vi "Main.vi"() -> ()   [LabVIEW 2017]
uses:
  1. CTL/State.ctl
  <vilib>/Utility/sysdir.llb/System Directory Type.ctl
  <vilib>/Instr/_visa.llb/VISA Configure Serial Port (Instr).vi
panel:
  in  "탭 컨트롤":enum32{"SETTING", "MAIN"}(tab)
  in  "로그인":bool
  in  "비밀번호":string
  in  "ID":string
  in  "COM포트":bool=TRUE
  in  "정지 버튼":bool=TRUE
  in  "PNF ON":bool=TRUE
  in  "데이터 저장":bool=TRUE
  out "시험결과":string
  out "1회시험결과":string
  out "2회시험결과":string
  out "3회시험결과":string
  out "String":string
  out "String 2":string
  out "String 3":string
  in  "VISA resource name":refnum<visa-resource-name> caption="VISA 리소스 이름"
  in  "Radio Buttons":enum32{"Item 0", "Item 1"}(radio)
  # "GUI Setting(KWFI)"
  # "ID"
  # "password"
  # "AUV Pinger TEST"
  # "음파발생기 TEST"
  # "시험 결과"
  # "시험 결과"
  # "1회 시험 데이터"
  # "2회 시험 데이터"
  # "3회 시험 데이터"
  # "1회 시험 결과"
  # "2회 시험 결과"
  # "3회 시험 결과"
  # "1회 시험 결과"
  # "2회 시험 결과"
  # "3회 시험 결과"
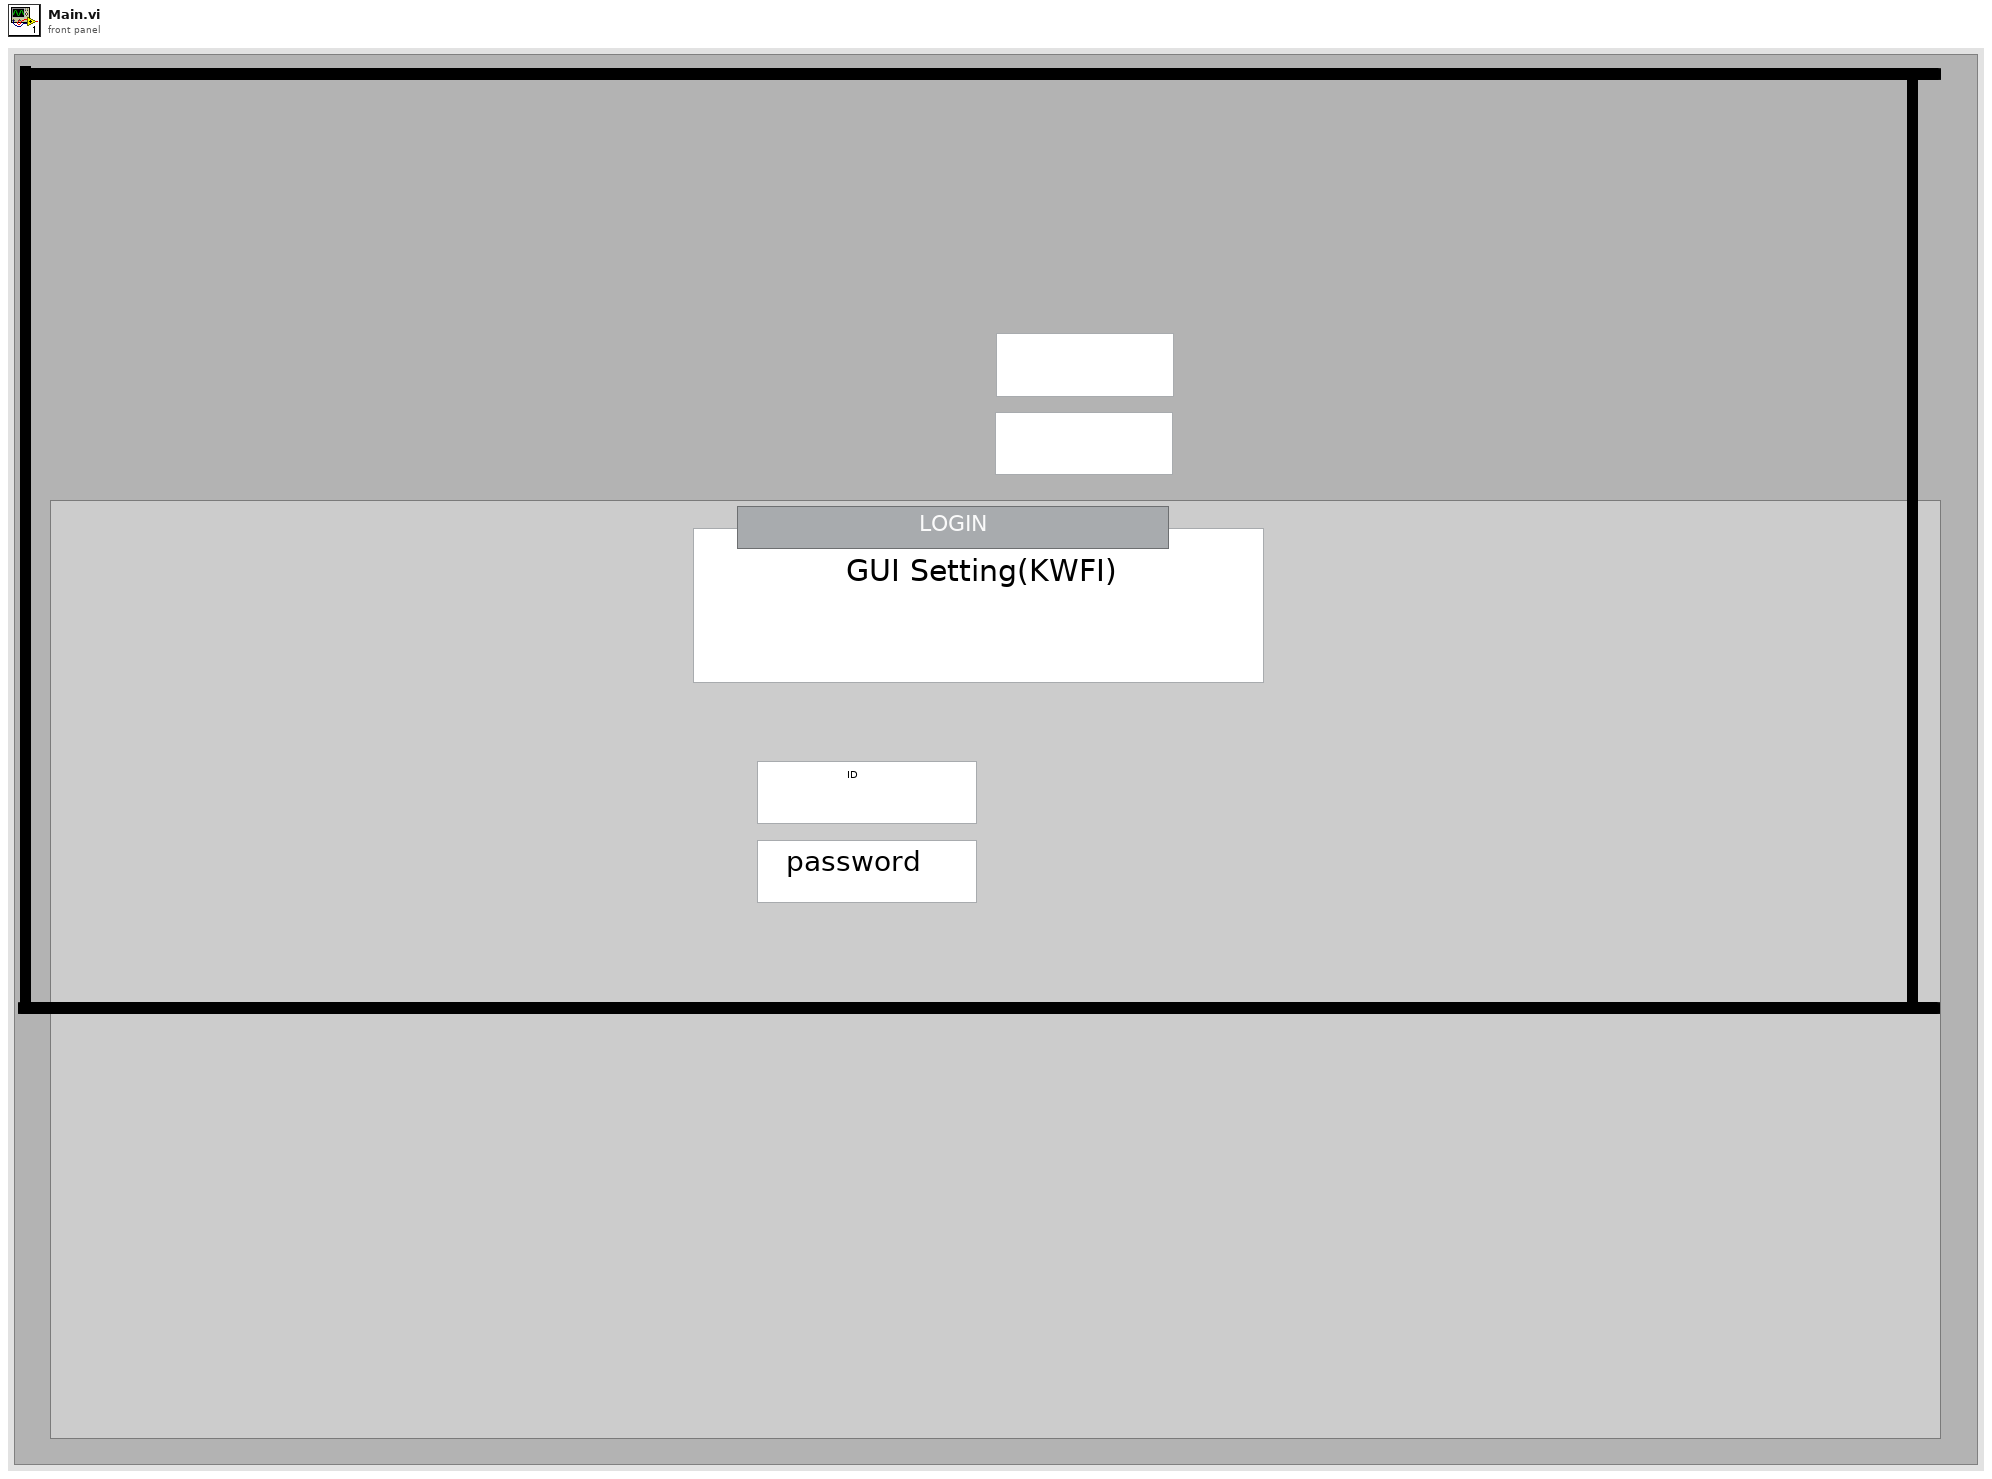
[diagram p1: front panel]
types:
  T1 = cluster{"1회 시험결과":string, "2회 시험결과":string, "3회 시험결과":string, "시험결과":string, "COM 포트":refnum<visa-resource-name>, "카운터":i32, "1회 로그":string, "2회 로그":string, "3회 로그":string, "1회 결과 카운트":i32, "2회 결과 카운트":i32, "3회 결과 카운트":i32, "관리자모드":bool, "1회 데이터":string[], "2회 데이터":string[], "3회 데이터":string[]}
  T2 = typedef "State.ctl" = enum16{"초기화", "시작", "정지", "데이터 저장", "로그인"}
  T3 = enum16{"open", "open or create", "create or replace", "create", "open (read-only)"}
  T4 = typedef "System Directory Type.ctl" = i32
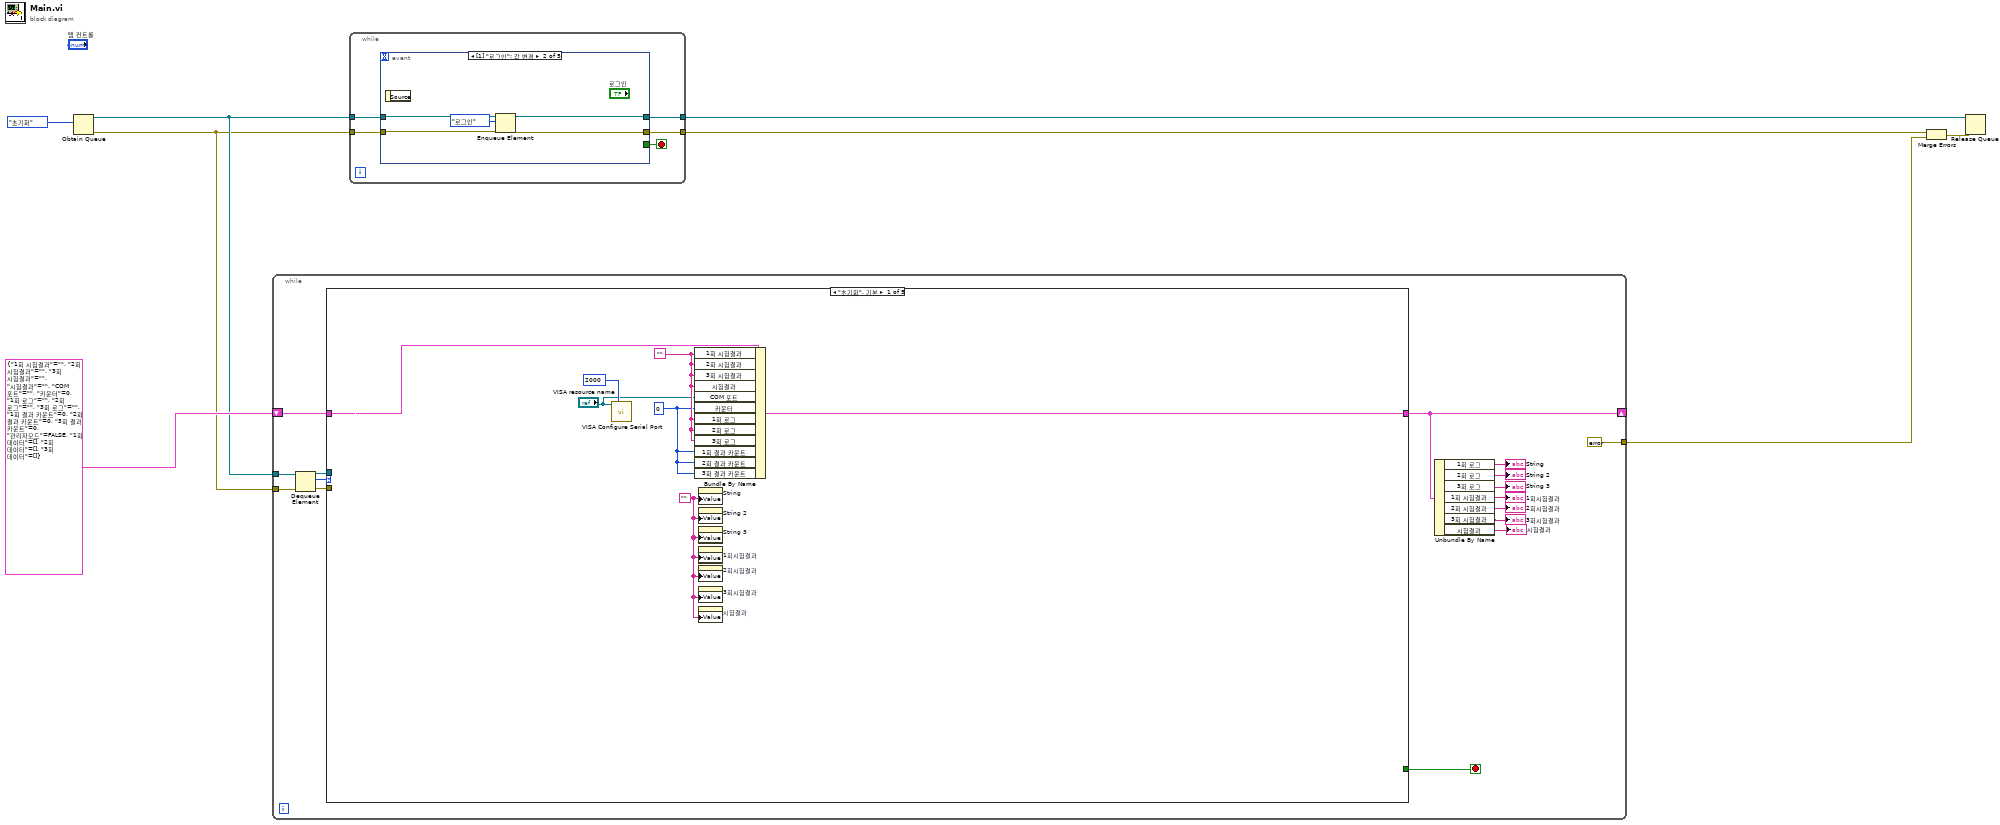
[diagram p0: block diagram]
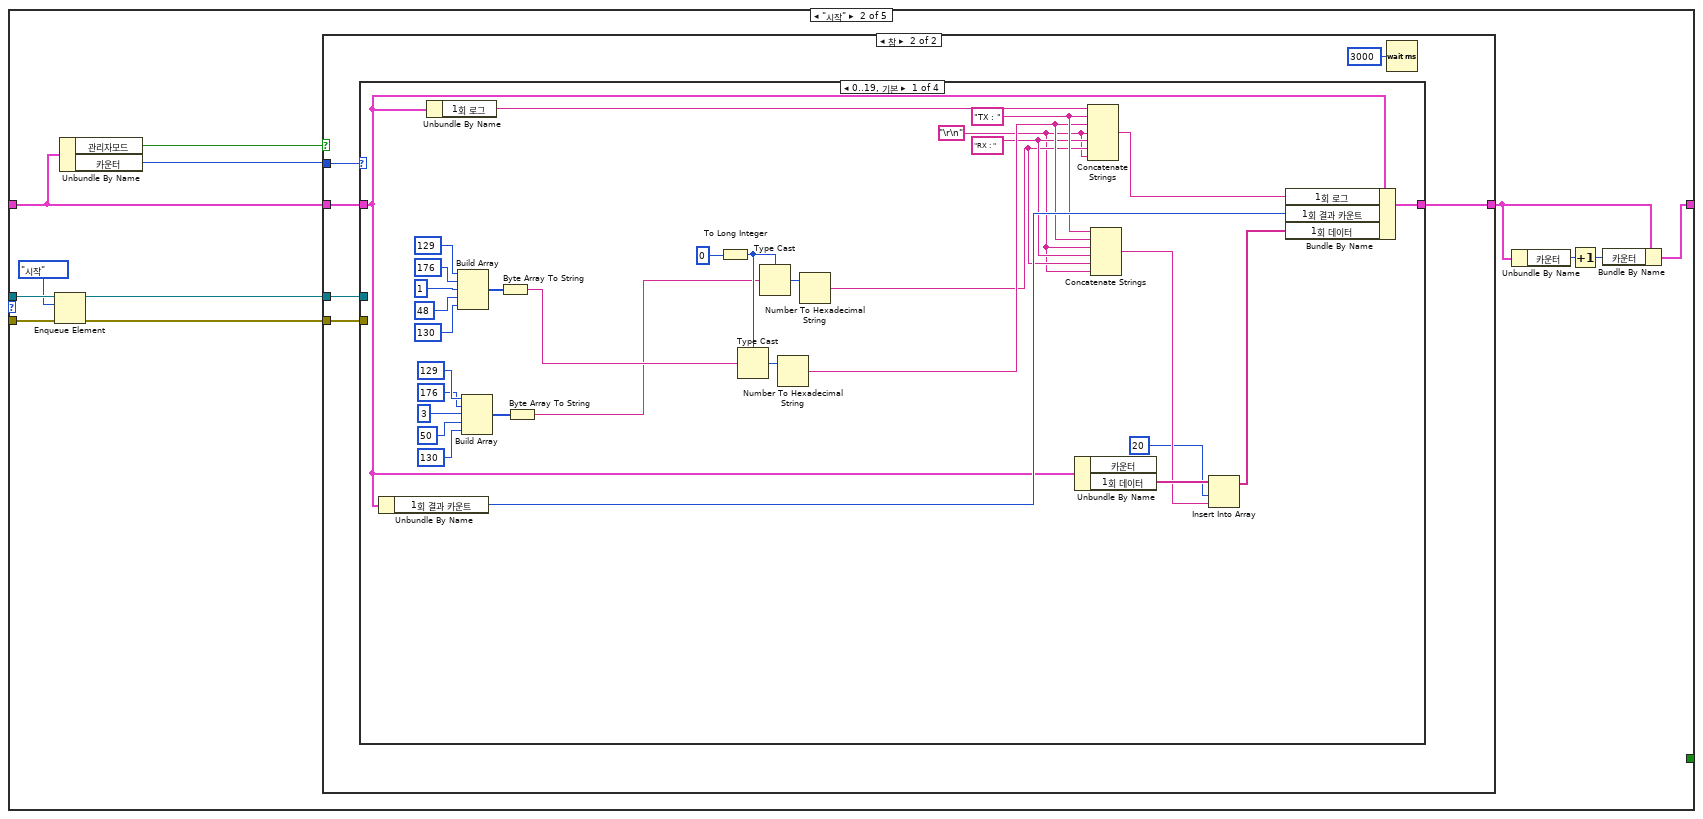
[diagram p2: hidden frame]
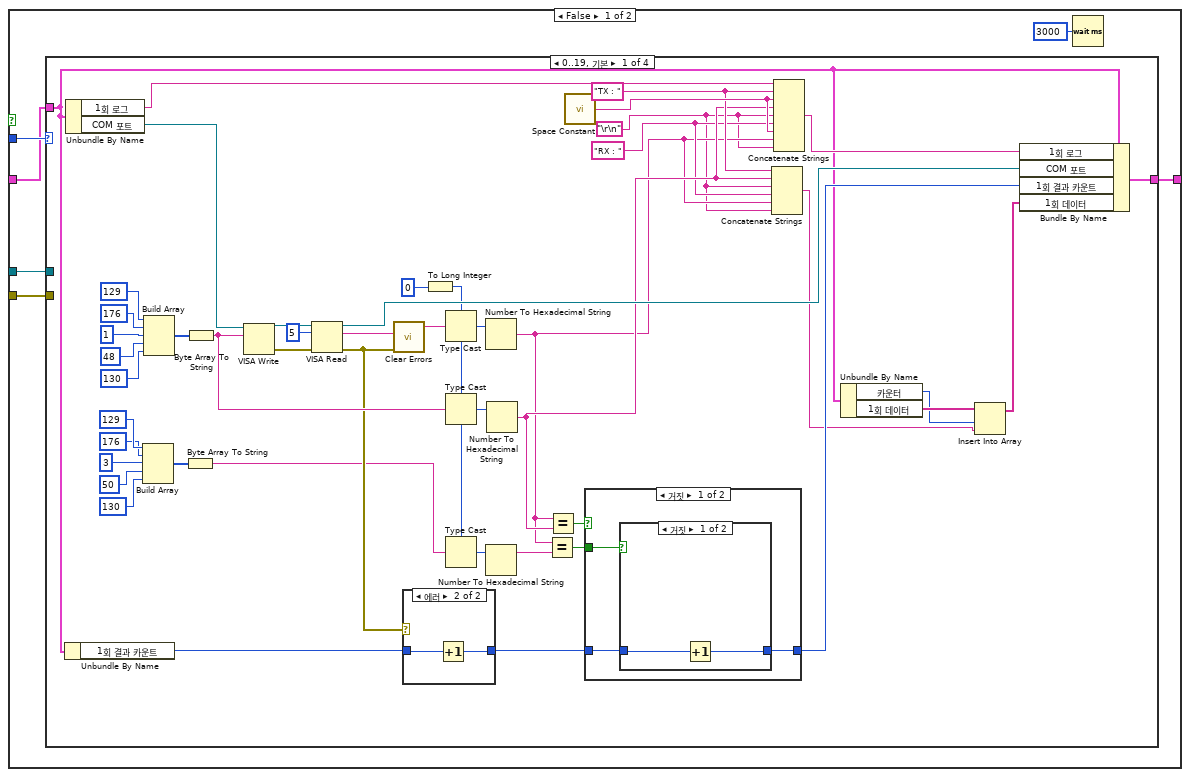
[diagram p3: hidden frame]
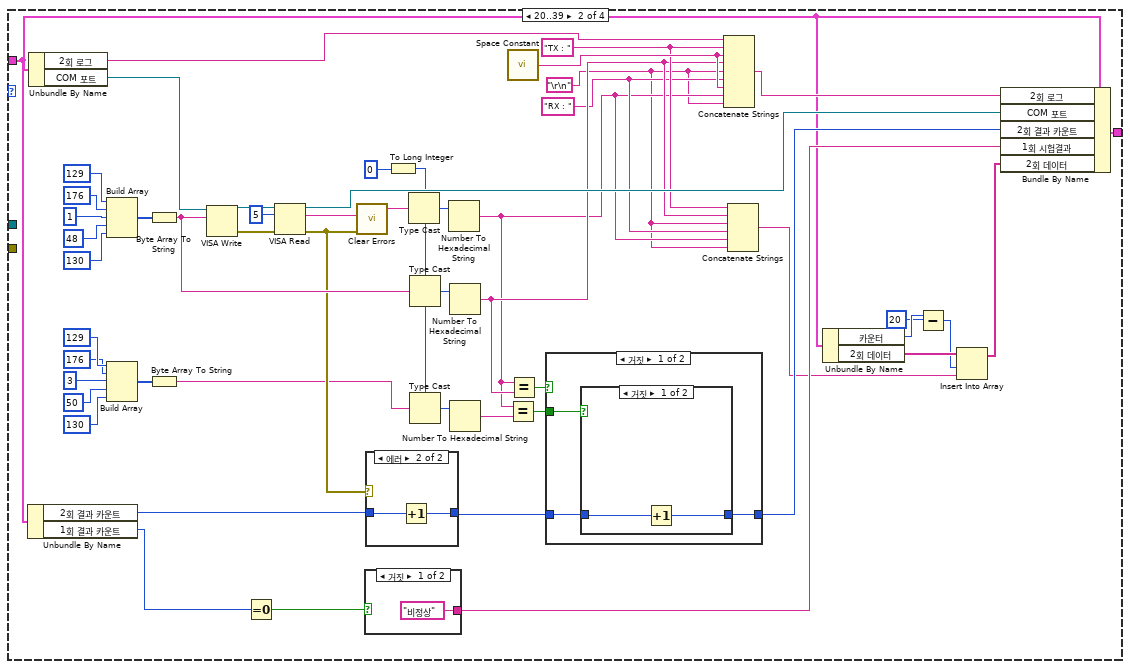
[diagram p7: hidden frame]
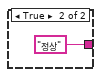
[diagram p10: hidden frame]
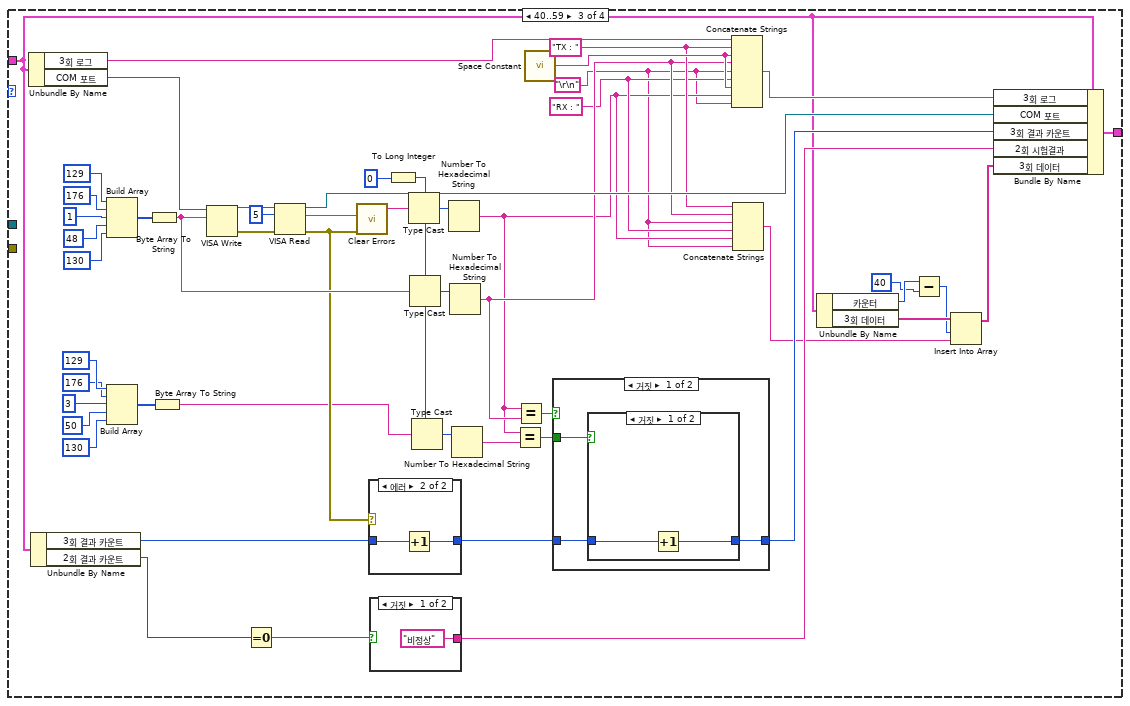
[diagram p12: hidden frame]
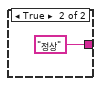
[diagram p15: hidden frame]
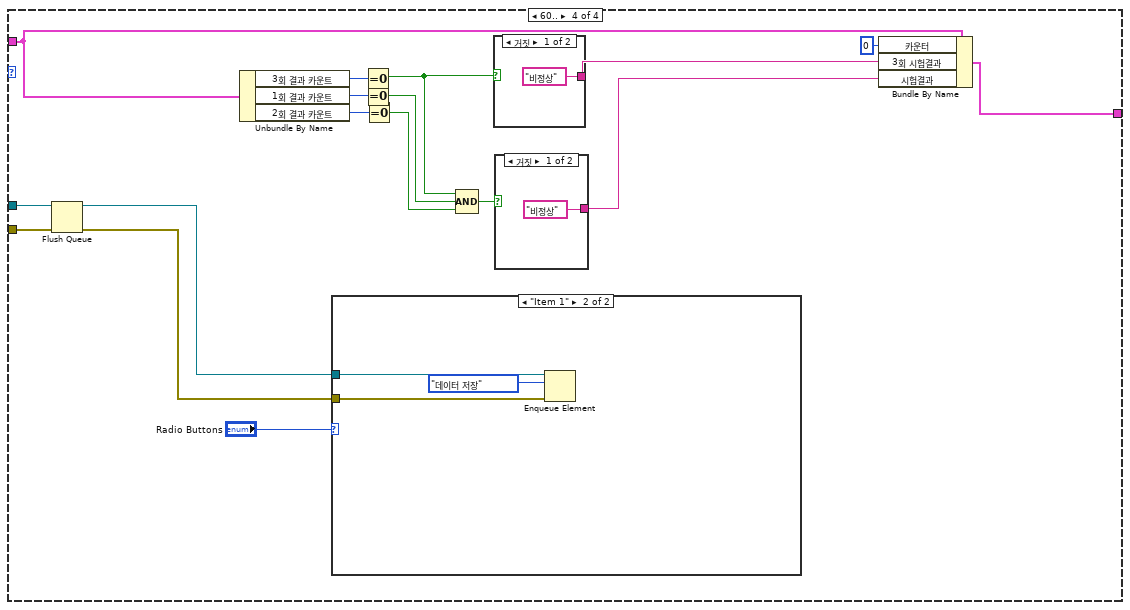
[diagram p17: hidden frame]
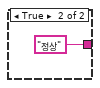
[diagram p19: hidden frame]
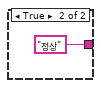
[diagram p20: hidden frame]
diagram:
  n1 = Obtain Queue(element data type=State."초기화") -> (queue out=w2:refnum<queue>, error out=w1:errorcluster)  [unwired: 4 in, 1 out]
  n2 = while {
    tunnel: w2 -> [w20]
    tunnel: w1 -> [w24]
    tunnel: [errorcluster {"status"=FALSE, "code"=0, "source"=""} ("에러 상수")] -> w6
    shift-right: [w9] -> _
    shift-left: T1 {"1회 시험결과"="", "2회 시험결과"="", "3회 시험결과"="", "시험결과"="", "COM 포트"="", "카운터"=0, "1회 로그"="", "2회 로그"="", "3회 로그"="", "1회 결과 카운트"=0, "2회 결과 카운트"=0, "3회 결과 카운트"=0, "관리자모드"=FALSE, "1회 데이터"=[], "2회 데이터"=[], "3회 데이터"=[]} -> [w21]
    stop <- w23 stop-if-true
    n3 = Dequeue Element(queue=w20, error in (no error)=w24) -> (queue out=w18:refnum<queue>, element=w19:T2, error out=w17:errorcluster)  [unwired: 1 in, 1 out]
    n4 = case shown="\"초기화\", 기본" w19 {
      tunnel: [_ _ TRUE _ _] -> w23
      tunnel: w21 -> [w31 w36 w386 w406 w440]
      tunnel: w18 -> [_ w42 _ w430 _]
      tunnel: w17 -> [_ w41 _ w429 _]
      tunnel: [w27 w32 w386 w406 w439] -> w9
      frame "초기화", Default {
        w28 = 0
        w29 = ""
        w30 = ""
        n5 = call-poly "VISA Configure Serial Port"("VISA resource name"="VISA resource name", "timeout (10sec)"=u32 2000) -> ()  [unwired: 12 in, 2 out]
        n6 = Bundle By Name(cluster=w31, "1회 시험결과"=w29, "2회 시험결과"=w29, "3회 시험결과"=w29, "시험결과"=w29, "COM 포트"="VISA resource name", "카운터"=w28, "1회 로그"=w29, "2회 로그"=w29, "3회 로그"=w29, "1회 결과 카운트"=w28, "2회 결과 카운트"=w28, "3회 결과 카운트"=w28) -> (w27:T1)
        n7 = property on="String" class="Str"("Value"=w30) -> ()  [unwired: 2 in, 2 out]
        n8 = property on="String 2" class="Str"("Value"=w30) -> ()  [unwired: 2 in, 2 out]
        n9 = property on="String 3" class="Str"("Value"=w30) -> ()  [unwired: 2 in, 2 out]
        n10 = property on="1회시험결과" class="Str"("Value"=w30) -> ()  [unwired: 2 in, 2 out]
        n11 = property on="2회시험결과" class="Str"("Value"=w30) -> ()  [unwired: 2 in, 2 out]
        n12 = property on="3회시험결과" class="Str"("Value"=w30) -> ()  [unwired: 2 in, 2 out]
        n13 = property on="시험결과" class="Str"("Value"=w30) -> ()  [unwired: 2 in, 2 out]
      }
      frame "시작" {
        n14 = Enqueue Element(queue=w42, element=State."시작", error in (no error)=w41) -> (queue out=w39:refnum<queue>, error out=w38:errorcluster)  [unwired: 1 in, 1 out]
        n15 = Unbundle By Name(w36) -> ("관리자모드"=w37:bool, "카운터"=w43:i32)
        n16 = case shown="참" w37 {
          tunnel: w43 -> [w49 w261]
          tunnel: w39 -> [w48 w260]
          tunnel: w38 -> [w47 w259]
          tunnel: [w45 w257] -> w33
          tunnel: w36 -> [w44 w256]
          frame False {
            n17 = case shown="0..19, 기본" w49 {
              tunnel: w44 -> [w54 w116 w179 w246]
              tunnel: [w95 w156 w219 w247] -> w45
              tunnel: w48 -> [_ _ _ w243]
              tunnel: w47 -> [_ _ _ w242]
              frame 0..19, Default {
                w57 = "RX : "
                w55 = "\r\n"
                w59 = "TX : "
                n18 = Unbundle By Name(w54) -> ("1회 결과 카운트"=w76:i32)
                n19 = Unbundle By Name(w54) -> ("1회 로그"=w82:string, "COM 포트"=w81:refnum<visa-resource-name>)
                n20 = Build Array(129, 176, 3, 50, 130) -> (w74:i32[])
                n21 = Build Array(129, 176, 1, 48, 130) -> (w86:i32[])
                n22 = Byte Array To String(unsigned byte array=w74) -> (string=w67:string)
                n23 = Byte Array To String(unsigned byte array=w86) -> (string=w80:string)
                n24 = VISA Write(VISA resource name=w81, write buffer=w80) -> (VISA resource name out=w94:refnum<visa-resource-name>, error out=w92:errorcluster)  [unwired: 1 in, 1 out]
                n25 = VISA Read(VISA resource name=w94, byte count=u32 5 ("바이트 카운트"), error in (no error)=w92) -> (VISA resource name out=w79:refnum<visa-resource-name>, read buffer=w85:string, error out=w77:errorcluster)  [unwired: 1 out]
                n26 = call <vilib>:"Clear Errors.vi"("error in (no error)"=w77) -> ()  [unwired: 5 in, 2 out]
                n27 = case shown="에러" w77 {
                  tunnel: [w103 w105] -> w63
                  tunnel: w76 -> [w103 w104]
                  frame No Error {
                  }
                  frame Error {
                    n28 = Increment(x=w104) -> (x+1=w105:i32)
                  }
                }
                n29 = To Long Integer(number=0 ("숫자")) -> (32bit integer=w68:i32)
                n30 = Type Cast(type=w68, x=w85) -> (*(type *) &x=w84:i32)
                n31 = Type Cast(type=w68, x=w80) -> (*(type *) &x=w78:i32)
                n32 = Type Cast(type=w68, x=w67) -> (*(type *) &x=w66:i32)
                n33 = Number To Hexadecimal String(2:w84) -> (0:w56:string)  [unwired: 1 in]
                n34 = Number To Hexadecimal String(2:w66) -> (0:w64:string)  [unwired: 1 in]
                n35 = Number To Hexadecimal String(2:w78) -> (0:w58:string)  [unwired: 1 in]
                n36 = Equal?(x=w56, y=w64) -> (x = y?=w65:bool)
                n37 = Equal?(x=w56, y=w58) -> (x = y?=w75:bool)
                n38 = call <vilib>:"Space Constant.vi"() -> ("String"=w61:string)
                n39 = case shown="거짓" w75 {
                  tunnel: w65 -> [w98 _]
                  tunnel: w63 -> [w97 w102]
                  tunnel: [w96 w102] -> w62
                  frame False {
                    n40 = case shown="거짓" w98 {
                      tunnel: w97 -> [w100 w101]
                      tunnel: [w99 w101] -> w96
                      frame False {
                        n41 = Increment(x=w100) -> (x+1=w99:i32)
                      }
                      frame True {
                      }
                    }
                  }
                  frame True {
                  }
                }
                n42 = Concatenate Strings(w59, w58, w55, w57, w56, w55) -> (w52:string)
                n43 = Concatenate Strings(w82, w59, w61, w58, w55, w57, w61, w56, w55) -> (w60:string)
                n44 = Unbundle By Name(w54) -> ("카운터"=w50:i32, "1회 데이터"=w53:string[])
                n45 = Insert Into Array(array=w53, index=w50, new element=w52) -> (w51:string[])
                n46 = Bundle By Name(cluster=w54, "1회 로그"=w60, "COM 포트"=w79, "1회 결과 카운트"=w62, "1회 데이터"=w51) -> (w95:T1)
              }
              frame 20..39 {
                w113 = "RX : "
                w111 = "\r\n"
                w115 = "TX : "
                n47 = Unbundle By Name(w116) -> ("2회 결과 카운트"=w138:i32, "1회 결과 카운트"=w137:i32)
                n48 = Unbundle By Name(w116) -> ("2회 로그"=w120:string, "COM 포트"=w143:refnum<visa-resource-name>)
                n49 = Build Array(129, 176, 1, 48, 130) -> (w147:i32[])
                n50 = Build Array(129, 176, 3, 50, 130) -> (w132:i32[])
                n51 = Byte Array To String(unsigned byte array=w147) -> (string=w142:string)
                n52 = Byte Array To String(unsigned byte array=w132) -> (string=w124:string)
                n53 = VISA Write(VISA resource name=w143, write buffer=w142) -> (VISA resource name out=w155:refnum<visa-resource-name>, error out=w153:errorcluster)  [unwired: 1 in, 1 out]
                n54 = Equal To 0?(x=w137) -> (x = 0?=w136:bool)
                n55 = VISA Read(VISA resource name=w155, byte count=u32 5 ("바이트 카운트"), error in (no error)=w153) -> (VISA resource name out=w141:refnum<visa-resource-name>, read buffer=w146:string, error out=w139:errorcluster)  [unwired: 1 out]
                n56 = call <vilib>:"Clear Errors.vi"("error in (no error)"=w139) -> ()  [unwired: 5 in, 2 out]
                n57 = case shown="거짓" w136 {
                  tunnel: ["비정상" "정상"] -> w135
                  frame False {
                  }
                  frame True {
                  }
                }
                n58 = case shown="에러" w139 {
                  tunnel: [w166 w168] -> w122
                  tunnel: w138 -> [w166 w167]
                  frame No Error {
                  }
                  frame Error {
                    n59 = Increment(x=w167) -> (x+1=w168:i32)
                  }
                }
                n60 = To Long Integer(number=0 ("숫자")) -> (32bit integer=w125:i32)
                n61 = Type Cast(type=w125, x=w146) -> (*(type *) &x=w145:i32)
                n62 = Type Cast(type=w125, x=w142) -> (*(type *) &x=w140:i32)
                n63 = Type Cast(type=w125, x=w124) -> (*(type *) &x=w126:i32)
                n64 = Number To Hexadecimal String(2:w145) -> (0:w112:string)  [unwired: 1 in]
                n65 = Number To Hexadecimal String(2:w140) -> (0:w114:string)  [unwired: 1 in]
                n66 = Number To Hexadecimal String(2:w126) -> (0:w123:string)  [unwired: 1 in]
                n67 = call <vilib>:"Space Constant.vi"() -> ("String"=w119:string)
                n68 = Equal?(x=w112, y=w123) -> (x = y?=w133:bool)
                n69 = Equal?(x=w112, y=w114) -> (x = y?=w134:bool)
                n70 = case shown="거짓" w134 {
                  tunnel: w133 -> [w159 _]
                  tunnel: w122 -> [w158 w163]
                  tunnel: [w157 w163] -> w121
                  frame False {
                    n71 = case shown="거짓" w159 {
                      tunnel: w158 -> [w161 w162]
                      tunnel: [w160 w162] -> w157
                      frame False {
                        n72 = Increment(x=w161) -> (x+1=w160:i32)
                      }
                      frame True {
                      }
                    }
                  }
                  frame True {
                  }
                }
                n73 = Concatenate Strings(w120, w115, w119, w114, w111, w113, w119, w112, w111) -> (w118:string)
                n74 = Concatenate Strings(w115, w114, w111, w113, w112, w111) -> (w110:string)
                n75 = Unbundle By Name(w116) -> ("카운터"=w108:i32, "2회 데이터"=w117:string[])
                n76 = Subtract(x=w108, y=20) -> (x-y=w106:i32)
                n77 = Insert Into Array(array=w117, index=w106, new element=w110) -> (w109:string[])
                n78 = Bundle By Name(cluster=w116, "2회 로그"=w118, "COM 포트"=w141, "2회 결과 카운트"=w121, "1회 시험결과"=w135, "2회 데이터"=w109) -> (w156:T1)
              }
              frame 40..59 {
                w176 = "RX : "
                w174 = "\r\n"
                w178 = "TX : "
                n79 = Unbundle By Name(w179) -> ("3회 로그"=w183:string, "COM 포트"=w206:refnum<visa-resource-name>)
                n80 = Unbundle By Name(w179) -> ("3회 결과 카운트"=w201:i32, "2회 결과 카운트"=w200:i32)
                n81 = Build Array(129, 176, 1, 48, 130) -> (w210:i32[])
                n82 = Build Array(129, 176, 3, 50, 130) -> (w195:i32[])
                n83 = Byte Array To String(unsigned byte array=w210) -> (string=w205:string)
                n84 = Byte Array To String(unsigned byte array=w195) -> (string=w187:string)
                n85 = VISA Write(VISA resource name=w206, write buffer=w205) -> (VISA resource name out=w218:refnum<visa-resource-name>, error out=w216:errorcluster)  [unwired: 1 in, 1 out]
                n86 = Equal To 0?(x=w200) -> (x = 0?=w199:bool)
                n87 = VISA Read(VISA resource name=w218, byte count=u32 5 ("바이트 카운트"), error in (no error)=w216) -> (VISA resource name out=w204:refnum<visa-resource-name>, read buffer=w209:string, error out=w202:errorcluster)  [unwired: 1 out]
                n88 = call <vilib>:"Clear Errors.vi"("error in (no error)"=w202) -> ()  [unwired: 5 in, 2 out]
                n89 = case shown="에러" w202 {
                  tunnel: [w229 w231] -> w185
                  tunnel: w201 -> [w229 w230]
                  frame No Error {
                  }
                  frame Error {
                    n90 = Increment(x=w230) -> (x+1=w231:i32)
                  }
                }
                n91 = case shown="거짓" w199 {
                  tunnel: ["비정상" "정상"] -> w198
                  frame False {
                  }
                  frame True {
                  }
                }
                n92 = To Long Integer(number=0 ("숫자")) -> (32bit integer=w188:i32)
                n93 = Type Cast(type=w188, x=w209) -> (*(type *) &x=w208:i32)
                n94 = Type Cast(type=w188, x=w205) -> (*(type *) &x=w203:i32)
                n95 = Type Cast(type=w188, x=w187) -> (*(type *) &x=w189:i32)
                n96 = Number To Hexadecimal String(2:w208) -> (0:w175:string)  [unwired: 1 in]
                n97 = Number To Hexadecimal String(2:w203) -> (0:w177:string)  [unwired: 1 in]
                n98 = Number To Hexadecimal String(2:w189) -> (0:w186:string)  [unwired: 1 in]
                n99 = Equal?(x=w175, y=w186) -> (x = y?=w196:bool)
                n100 = Equal?(x=w175, y=w177) -> (x = y?=w197:bool)
                n101 = call <vilib>:"Space Constant.vi"() -> ("String"=w182:string)
                n102 = case shown="거짓" w197 {
                  tunnel: w196 -> [w222 _]
                  tunnel: w185 -> [w221 w226]
                  tunnel: [w220 w226] -> w184
                  frame False {
                    n103 = case shown="거짓" w222 {
                      tunnel: w221 -> [w224 w225]
                      tunnel: [w223 w225] -> w220
                      frame False {
                        n104 = Increment(x=w224) -> (x+1=w223:i32)
                      }
                      frame True {
                      }
                    }
                  }
                  frame True {
                  }
                }
                n105 = Concatenate Strings(w183, w178, w182, w177, w174, w176, w182, w175, w174) -> (w181:string)
                n106 = Concatenate Strings(w178, w177, w174, w176, w175, w174) -> (w173:string)
                n107 = Unbundle By Name(w179) -> ("카운터"=w171:i32, "3회 데이터"=w180:string[])
                n108 = Subtract(x=w171, y=40) -> (x-y=w169:i32)
                n109 = Insert Into Array(array=w180, index=w169, new element=w173) -> (w172:string[])
                n110 = Bundle By Name(cluster=w179, "3회 로그"=w181, "COM 포트"=w204, "3회 결과 카운트"=w184, "2회 시험결과"=w198, "3회 데이터"=w172) -> (w219:T1)
              }
              frame 60.. {
                n111 = Flush Queue(queue=w243, error in (no error)=w242) -> (queue out=w233:refnum<queue>, error out=w232:errorcluster)  [unwired: 1 out]
                n112 = Unbundle By Name(w246) -> ("3회 결과 카운트"=w245:i32, "1회 결과 카운트"=w241:i32, "2회 결과 카운트"=w240:i32)
                n113 = case shown="\"Item 1\"" "Radio Buttons" {
                  tunnel: w233 -> [_ w251]
                  tunnel: w232 -> [_ w250]
                  frame "Item 0", Default {
                  }
                  frame "Item 1" {
                    n114 = Enqueue Element(queue=w251, element=State."데이터 저장", error in (no error)=w250) -> ()  [unwired: 1 in, 3 out]
                  }
                }
                n115 = Equal To 0?(x=w245) -> (x = 0?=w239:bool)
                n116 = Equal To 0?(x=w241) -> (x = 0?=w238:bool)
                n117 = Equal To 0?(x=w240) -> (x = 0?=w237:bool)
                n118 = Compound Arithmetic op=AND(w239, w238, w237) -> (w236:bool)
                n119 = case shown="거짓" w239 {
                  tunnel: ["비정상" "정상"] -> w244
                  frame False {
                  }
                  frame True {
                  }
                }
                n120 = case shown="거짓" w236 {
                  tunnel: ["비정상" "정상"] -> w235
                  frame False {
                  }
                  frame True {
                  }
                }
                n121 = Bundle By Name(cluster=w246, "카운터"=0, "3회 시험결과"=w244, "시험결과"=w235) -> (w247:T1)
              }
            }
            n122 = Wait (ms)(milliseconds to wait=u32 3000 ("대기 시간 (ms)")) -> ()  [unwired: 1 out]
          }
          frame True {
            n123 = case shown="0..19, 기본" w261 {
              tunnel: w256 -> [w264 w297 w336 w377]
              tunnel: [w292 w329 w368 w378] -> w257
              tunnel: w260 -> [_ _ _ w373]
              tunnel: w259 -> [_ _ _ w372]
              frame 0..19, Default {
                w268 = "RX : "
                w270 = "TX : "
                w266 = "\r\n"
                n124 = Unbundle By Name(w264) -> ("1회 결과 카운트"=w279:i32)
                n125 = Unbundle By Name(w264) -> ("1회 로그"=w283:string)
                n126 = Build Array(129, 176, 1, 48, 130) -> (w286:i32[])
                n127 = Build Array(129, 176, 3, 50, 130) -> (w278:i32[])
                n128 = Byte Array To String(unsigned byte array=w286) -> (string=w280:string)
                n129 = Byte Array To String(unsigned byte array=w278) -> (string=w272:string)
                n130 = To Long Integer(number=0 ("숫자")) -> (32bit integer=w282:i32)
                n131 = Type Cast(type=w282, x=w280) -> (*(type *) &x=w281:i32)
                n132 = Type Cast(type=w282, x=w272) -> (*(type *) &x=w285:i32)
                n133 = Number To Hexadecimal String(2:w281) -> (0:w269:string)  [unwired: 1 in]
                n134 = Number To Hexadecimal String(2:w285) -> (0:w267:string)  [unwired: 1 in]
                n135 = Unbundle By Name(w264) -> ("1회 데이터"=w271:string[])  [unwired: 1 out]
                n136 = Concatenate Strings(w283, w270, w269, w266, w268, w267, w266) -> (w293:string)
                n137 = Concatenate Strings(w270, w269, w266, w268, w267, w266) -> (w265:string)
                n138 = Insert Into Array(array=w271, index=20, new element=w265) -> (w263:string[])
                n139 = Bundle By Name(cluster=w264, "1회 로그"=w293, "1회 결과 카운트"=w279, "1회 데이터"=w263) -> (w292:T1)
              }
              frame 20..39 {
                w302 = "RX: "
                w304 = "TX: "
                w300 = "\r\n"
                n140 = Unbundle By Name(w297) -> ("2회 결과 카운트"=w314:i32, "1회 결과 카운트"=w317:i32)
                n141 = Unbundle By Name(w297) -> ("2회 로그"=w320:string)
                n142 = Build Array(129, 176, 3, 50, 130) -> (w312:i32[])
                n143 = Build Array(129, 176, 1, 48, 130) -> (w323:i32[])
                n144 = Byte Array To String(unsigned byte array=w323) -> (string=w313:string)
                n145 = Byte Array To String(unsigned byte array=w312) -> (string=w306:string)
                n146 = Equal To 0?(x=w317) -> (x = 0?=w316:bool)
                n147 = case shown="거짓" w316 {
                  tunnel: ["비정상" "정상"] -> w315
                  frame False {
                  }
                  frame True {
                  }
                }
                n148 = To Long Integer(number=0 ("숫자")) -> (32bit integer=w319:i32)
                n149 = Type Cast(type=w319, x=w306) -> (*(type *) &x=w322:i32)
                n150 = Type Cast(type=w319, x=w313) -> (*(type *) &x=w318:i32)
                n151 = Number To Hexadecimal String(2:w322) -> (0:w301:string)  [unwired: 1 in]
                n152 = Number To Hexadecimal String(2:w318) -> (0:w303:string)  [unwired: 1 in]
                n153 = Unbundle By Name(w297) -> ("카운터"=w296:i32, "2회 데이터"=w305:string[])
                n154 = Concatenate Strings(w320, w304, w303, w300, w302, w301, w300) -> (w330:string)
                n155 = Concatenate Strings(w304, w303, w300, w302, w301, w300) -> (w299:string)
                n156 = Subtract(x=w296, y=20) -> (x-y=w294:i32)
                n157 = Insert Into Array(array=w305, index=w294, new element=w299) -> (w298:string[])
                n158 = Bundle By Name(cluster=w297, "2회 로그"=w330, "2회 결과 카운트"=w314, "1회 시험결과"=w315, "2회 데이터"=w298) -> (w329:T1)
              }
              frame 40..59 {
                w341 = "RX: "
                w343 = "TX: "
                w339 = "\r\n"
                n159 = Unbundle By Name(w336) -> ("3회 결과 카운트"=w353:i32, "2회 결과 카운트"=w356:i32)
                n160 = Unbundle By Name(w336) -> ("3회 로그"=w359:string)
                n161 = Build Array(129, 176, 3, 50, 130) -> (w351:i32[])
                n162 = Build Array(129, 176, 1, 48, 130) -> (w362:i32[])
                n163 = Byte Array To String(unsigned byte array=w351) -> (string=w345:string)
                n164 = Byte Array To String(unsigned byte array=w362) -> (string=w352:string)
                n165 = Equal To 0?(x=w356) -> (x = 0?=w355:bool)
                n166 = case shown="거짓" w355 {
                  tunnel: ["비정상" "정상"] -> w354
                  frame False {
                  }
                  frame True {
                  }
                }
                n167 = To Long Integer(number=0 ("숫자")) -> (32bit integer=w358:i32)
                n168 = Type Cast(type=w358, x=w345) -> (*(type *) &x=w361:i32)
                n169 = Type Cast(type=w358, x=w352) -> (*(type *) &x=w357:i32)
                n170 = Number To Hexadecimal String(2:w361) -> (0:w340:string)  [unwired: 1 in]
                n171 = Number To Hexadecimal String(2:w357) -> (0:w342:string)  [unwired: 1 in]
                n172 = Unbundle By Name(w336) -> ("카운터"=w335:i32, "3회 데이터"=w344:string[])
                n173 = Concatenate Strings(w359, w343, w342, w339, w341, w340, w339) -> (w369:string)
                n174 = Concatenate Strings(w343, w342, w339, w341, w340, w339) -> (w338:string)
                n175 = Subtract(x=w335, y=40) -> (x-y=w333:i32)
                n176 = Insert Into Array(array=w344, index=w333, new element=w338) -> (w337:string[])
                n177 = Bundle By Name(cluster=w336, "3회 로그"=w369, "3회 결과 카운트"=w353, "2회 시험결과"=w354, "3회 데이터"=w337) -> (w368:T1)
              }
              frame 60.. {
                n178 = Flush Queue(queue=w373, error in (no error)=w372) -> ()  [unwired: 3 out]
                n179 = Unbundle By Name(w377) -> ("3회 결과 카운트"=w376:i32)
                n180 = Equal To 0?(x=w376) -> (x = 0?=w375:bool)
                n181 = case shown="거짓" w375 {
                  tunnel: ["비정상" "정상"] -> w374
                  frame False {
                  }
                  frame True {
                  }
                }
                n182 = Bundle By Name(cluster=w377, "카운터"=0, "3회 시험결과"=w374, "시험결과"=w374) -> (w378:T1)
              }
            }
            n183 = Wait (ms)(milliseconds to wait=u32 3000 ("대기 시간 (ms)")) -> ()  [unwired: 1 out]
          }
        }
        n184 = Unbundle By Name(w33) -> ("카운터"=w35:i32)
        n185 = Increment(x=w35) -> (x+1=w34:i32)
        n186 = Bundle By Name(cluster=w33, "카운터"=w34) -> (w32:T1)
      }
      frame "정지" {
        w385 = refnum<visa-resource-name> refnum  # COM 포트
        w387 = ""
        n187 = Unbundle By Name(w386) -> ("COM 포트"=w383:refnum<visa-resource-name>)
        n188 = Equal?(x=w383, y=w385) -> (x = y?=w384:bool)
        n189 = case shown="거짓" w384 {
          tunnel: w383 -> [w390 _]
          frame False {
            n190 = VISA Close(VISA resource name=w390) -> ()  [unwired: 1 in, 1 out]
          }
          frame True {
          }
        }
        n191 = property on="로그인" class="Bool (엄격한)"("Value"=TRUE ("로그인")) -> ()  [unwired: 2 in, 2 out]
        n192 = property on="탭 컨트롤" class="TabCtl (엄격한)"("Value"=enum32{"SETTING", "MAIN"}."SETTING" ("탭 컨트롤")) -> ()  [unwired: 2 in, 2 out]
        n193 = property on="비밀번호" class="Str"("Value"=w387) -> ()  [unwired: 2 in, 2 out]
        n194 = property on="ID" class="Str"("Value"=w387) -> ()  [unwired: 2 in, 2 out]
      }
      frame "데이터 저장" {
        w410 = refnum<visa-resource-name> refnum  # COM 포트
        w427 = T4 1 items=["사용자 홈"=0, "사용자 데스크탑"=1, "사용자 문서"=2, "사용자 어플리케이션 데이터"=3, "사용자 환경"=4, "사용자 임시"=5, "퍼블릭 문서"=6, "퍼블릭 어플리케이션 데이터"=7, "퍼블릭 환경"=8, "퍼블릭 캐시"=13, "시스템 코어 라이브러리"=9, "시스템 설치된 라이브러리"=10, "어플리케이션 파일"=11, "부팅 볼륨 루트"=12] ("system directory type")
        n195 = Enqueue Element(queue=w430, element=State."초기화", error in (no error)=w429) -> ()  [unwired: 1 in, 3 out]
        n196 = Unbundle By Name(w406) -> ("시험결과"=w393:string, "1회 데이터"=w396:string[], "2회 데이터"=w395:string[], "3회 데이터"=w394:string[])
        n197 = Build Array(w393) -> (w392:string[])
        n198 = Build Array(w396, w395, w394, w392) -> (w391:string[][])
        n199 = call <vilib>:"Get System Directory.vi"("system directory type"=w427) -> ("system directory"=w426:path)  [unwired: 10 in]
        n200 = Get Date/Time String(want seconds? (F)=TRUE ("초 보이기? (거짓)")) -> (date string=w413:string, time string=w417:string)  [unwired: 2 in]
        n201 = Build Path(base path=w426, name or relative path="Data_log" ("이름 또는 상대 경로")) -> (appended path=w424:path)
        n202 = call <vilib>:"Check if File or Folder Exists.vi"("path"=w424) -> ("error out"=w421:errorcluster, "file or folder exists?"=w423:bool, "dup path"=w422:path)  [unwired: 8 in]
        n203 = Search and Replace String(replace all?=TRUE ("모두 대체? (거짓)"), input string=w417, search string=":" ("검색 문자열"), replace string="_" ("대체 문자열(\"\")")) -> (result string=w414:string)  [unwired: 4 in, 3 out]
        n204 = case shown="거짓" w423 {
          tunnel: w422 -> [w436 w438]
          tunnel: w421 -> [w435 w437]
          tunnel: [w434 w438] -> w420
          tunnel: [w433 w437] -> _
          frame False {
            n205 = Create Folder(path (use dialog)=w436, error in=w435) -> (created path=w434:path, error out=w433:errorcluster)  [unwired: 1 in, 1 out]
          }
          frame True {
          }
        }
        n206 = Concatenate Strings(w413, w414, "_log.csv") -> (w411:string)
        n207 = Build Path(base path=w420, name or relative path=w411) -> (appended path=w405:path)
        n208 = TDMS Open(10:T3."open or create" ("동작(0:open)"), 11:w405) -> (0:w402:errorcluster, 3:w403:refnum<k34>)  [unwired: 5 in]
        n209 = TDMS Write(0:w403, 5:"Data" ("그룹 이름 입력(제목없음)"), 7:string[] ["1회 로그", "2회 로그", "3회 로그", "최종시험결과"], 9:w391, 11:w402) -> (4:w401:refnum<k34>, 15:w400:errorcluster)  [unwired: 1 in, 2 out]
        n210 = Unbundle By Name(w406) -> ("COM 포트"=w408:refnum<visa-resource-name>)
        n211 = Equal?(x=w408, y=w410) -> (x = y?=w409:bool)
        n212 = TDMS Close(8:w400, 11:w401) -> (0:w399:errorcluster)  [unwired: 1 out]
        n213 = case shown="참" w409 {
          tunnel: w408 -> [w432 _]
          tunnel: [w431 _] -> w407
          frame False {
            n214 = VISA Close(VISA resource name=w432) -> (error out=w431:errorcluster)  [unwired: 1 in]
          }
          frame True {
          }
        }
        n215 = Merge Errors(w407, w399) -> ()  [unwired: 1 out]
      }
      frame "로그인" {
        n216 = Equal?(x="kwfi", y="ID") -> (x = y?=w448:bool)
        n217 = Equal?(x="1234", y="비밀번호") -> (x = y?=w451:bool)
        n218 = Equal?(x="7890", y="비밀번호") -> (x = y?=w450:bool)
        n219 = And(x=w448, y=w451) -> (x .and. y?=w444:bool)
        n220 = And(x=w448, y=w450) -> (x .and. y?=w443:bool)
        n221 = Or(x=w444, y=w443) -> (x .or. y?=w445:bool)
        n222 = case shown="참" w445 {
          tunnel: w443 -> [_ w464]
          tunnel: [_ w461] -> w441
          tunnel: [FALSE TRUE] -> w442
          frame False {
          }
          frame True {
            # "로그인 상태"
            # "관리자모드"
            n223 = Select(t=TRUE, s=w464, f=FALSE) -> (s? t:f=w461:bool)
          }
        }
        n224 = case shown="참" w442 {
          tunnel: w441 -> [_ w457]
          tunnel: w440 -> [w454 w458]
          tunnel: [w454 w456] -> w439
          frame False {
          }
          frame True {
            n225 = Bundle By Name(cluster=w458, "관리자모드"=w457) -> (w456:T1)
            n226 = property on="탭 컨트롤" class="TabCtl (엄격한)"("Value"=enum32{"SETTING", "MAIN"}."MAIN" ("탭 컨트롤")) -> ()  [unwired: 2 in, 2 out]
          }
        }
      }
    }
    n227 = Unbundle By Name(w9) -> ("1회 로그"=→"String":string, "2회 로그"=→"String 2":string, "3회 로그"=→"String 3":string, "1회 시험결과"=→"1회시험결과":string, "2회 시험결과"=→"2회시험결과":string, "3회 시험결과"=→"3회시험결과":string, "시험결과"=→"시험결과":string)
  }
  n228 = while {
    tunnel: w2 -> [w469]
    tunnel: w1 -> [w468]
    tunnel: [w466] -> w7
    tunnel: [w465] -> w4
    stop <- w467 stop-if-true
    n229 = event shown="[1] \"로그인\": 값 변경" {
      selector: _ -> [_ _ _ _ _]
      dyn-events: _ -> [_ _ _ _ _]
      timeout: _ -> [_ _ _ _ _]
      tunnel: w469 -> [w470 w482 w487 w492 w497]
      tunnel: w468 -> [w471 w479 w486 w491 w496]
      tunnel: [TRUE _ _ _ _] -> w467
      tunnel: [w475 w480 w484 w488 w493] -> w466
      tunnel: [w474 w481 w485 w489 w494] -> w465
      event "정지 버튼": Value Change {
        n230 = event-data() -> ()  [unwired: 1 in, 1 out]
        n231 = Flush Queue(queue=w470, error in (no error)=w471) -> (queue out=w473:refnum<queue>, error out=w472:errorcluster)  [unwired: 1 out]
        n232 = Enqueue Element(queue=w473, element=State."정지", error in (no error)=w472) -> (queue out=w474:refnum<queue>, error out=w475:errorcluster)  [unwired: 1 in, 1 out]
      }
      event "로그인": Value Change {
        n233 = event-data() -> ()  [unwired: 1 in, 1 out]
        n234 = Enqueue Element(queue=w482, element=State."로그인" ("원소"), error in (no error)=w479) -> (queue out=w481:refnum<queue>, error out=w480:errorcluster)  [unwired: 1 in, 1 out]
      }
      event "COM포트": Value Change {
        n235 = event-data() -> ()  [unwired: 1 in, 1 out]
        n236 = Enqueue Element(queue=w487, element=State."초기화" ("원소"), error in (no error)=w486) -> (queue out=w485:refnum<queue>, error out=w484:errorcluster)  [unwired: 1 in, 1 out]
      }
      event "PNF ON": Value Change {
        n237 = event-data() -> ()  [unwired: 1 in, 1 out]
        n238 = Enqueue Element(queue=w492, element=State."시작", error in (no error)=w491) -> (queue out=w489:refnum<queue>, error out=w488:errorcluster)  [unwired: 1 in, 1 out]
      }
      event "데이터 저장": Value Change {
        n239 = event-data() -> ()  [unwired: 1 in, 1 out]
        n240 = Enqueue Element(queue=w497, element=State."데이터 저장", error in (no error)=w496) -> (queue out=w494:refnum<queue>, error out=w493:errorcluster)  [unwired: 1 in, 1 out]
      }
    }
  }
  n241 = Merge Errors(w7, w6) -> (w5:errorcluster)
  n242 = Release Queue(queue=w4, error in (no error)=w5) -> ()  [unwired: 1 in, 3 out]
